vi "Save-Recall Settings.vi"(8 "error in (no error)":errorcluster, 9 "Action":enum16{"Save", "Recall"}(ring), 10 "Setting No.":u32, 11 "DG645 in":refnum<class "DG645.lvclass">) -> (0 "error out":errorcluster, 3 "DG645 out":refnum<class "DG645.lvclass">)   [LabVIEW 2018, in "DG645.lvlib" / "DG645.lvclass"]
uses:
  DG645.lvclass
  DG645.lvclass/DG645.ctl
  <instrlib>/Stanford Research DG645/Stanford Research DG645.lvlib
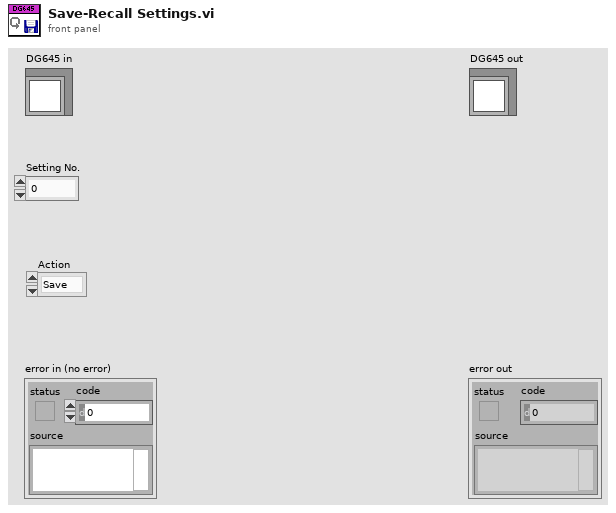
[diagram p1: front panel]
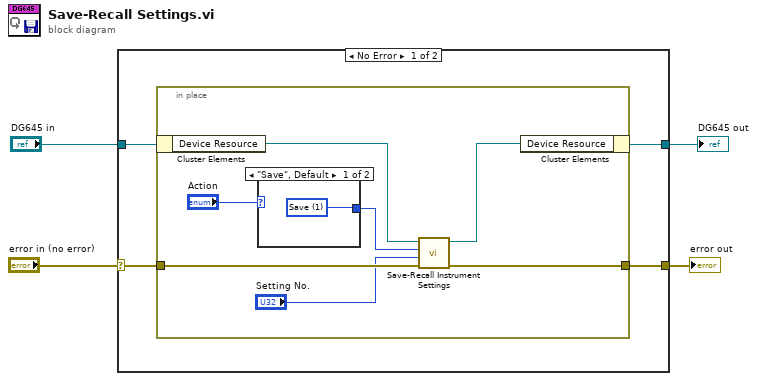
[diagram p0: block diagram]
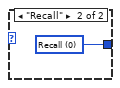
[diagram p2: hidden frame]
diagram:
  n1 = case shown="No Error" "error in (no error)" {
    selector: "error in (no error)" -> [w8 w19]
    tunnel: "DG645 in" -> [w7 w18]
    tunnel: [w6 w18] -> w2
    tunnel: [w5 w19] -> w1
    frame No Error {
      n2 = in-place {
        in-place-border: w8 -> [w14]
        in-place-border: [w9] -> w5
        n3 = in-place-cluster #1(w7) -> ("Device Resource"=w15:refnum<visa-resource-name>)
        n4 = case shown="\"Save\", Default" "Action" {
          tunnel: [w16 w17] -> w11
          frame "Save", Default {
            w16 = u16 1 items=["Recall", "Save"] ("Recall or Save (0:Recall)")
          }
          frame "Recall" {
            w17 = u16 0 items=["Recall", "Save"] ("Recall or Save (0:Recall)")
          }
        }
        n5 = call <instrlib>:"Save-Recall Instrument Settings.vi"("error in (no error)"=w14, "Save Number (0)"="Setting No.", "Recall or Save (0:Recall)"=w11, "VISA resource name"=w15) -> ("error out"=w9:errorcluster, "VISA resource name out"=w13:refnum<visa-resource-name>)  [unwired: 6 in]
        n6 = in-place-cluster #1("Device Resource"=w13) -> (w6:refnum<class "DG645.lvclass">)
      }
    }
    frame Error {
    }
  }
  "error out" <- w1
  "DG645 out" <- w2
